vi "PowerSupplyModule.vi"(8 "error in (no error)":errorcluster, 9 "Shutdown Event":refnum<user-event>, 10 "Config":T1, 11 "ModuleID":string) -> (0 "error out":errorcluster)   [LabVIEW 2020, in "PowerSupply.lvlib"]
uses:
  PowerSupply.lvlib
  <vilib>/Utility/Data Type/Type Definitions/Data Type.ctl
  <vilib>/Utility/Data Type/NI_Data Type.lvlib
  eac3c09b-8ce1-4b18-8db3-0e6b686db002.vi
  <vilib>/Tag Engine/Types/SetRequest Cluster.ctl
  <vilib>/Tag Engine/Tag Engine Core.lvlib
  5bc3bb94-1071-4bc4-bea8-59b69d9a0ea3.vi
  2c36721a-ae4d-497d-865d-af4d970190ac.vi
  e0a74cc3-df72-4da2-81c8-b90a0d719853.vi
  32760def-be6c-40d5-9cdc-91618a22e337.vi
  fa7b8413-0d77-4427-8bf4-75f68590801f.vi
  674e74a0-18a0-4cb1-b513-5d1b134eea45.vi
  <vilib>/Tag Engine/Tag/Tag.lvclass
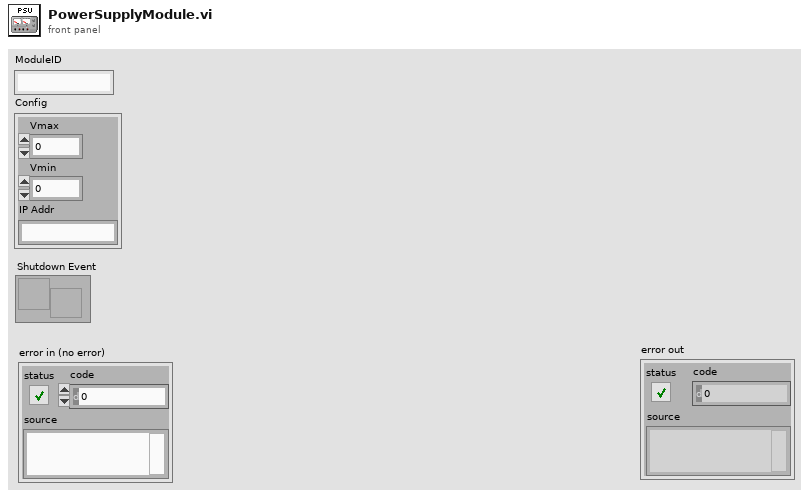
[diagram p1: front panel]
types:
  T1 = cluster{"Vmax":dbl, "Vmin":dbl, "IP Addr":string}
  T2 = cluster{"Config":cluster{"Vmax":dbl, "Vmin":dbl, "IP Addr":string}, "Tag Refs":cluster{"VOLT_SV":refnum<data-value>, "VOLT_PV":refnum<data-value>, "CURR_PV":refnum<data-value>, "OUTPUT_EN":refnum<data-value>}}
  T3 = cluster{"VOLT_SV":refnum<user-event>, "OUTPUT_EN":refnum<user-event>}
  T4 = cluster{"VOLT_SV":refnum<data-value>, "VOLT_PV":refnum<data-value>, "CURR_PV":refnum<data-value>, "OUTPUT_EN":refnum<data-value>}
  T5 = cluster{"Req Value":variant, "Callback":refnum<notifier>}
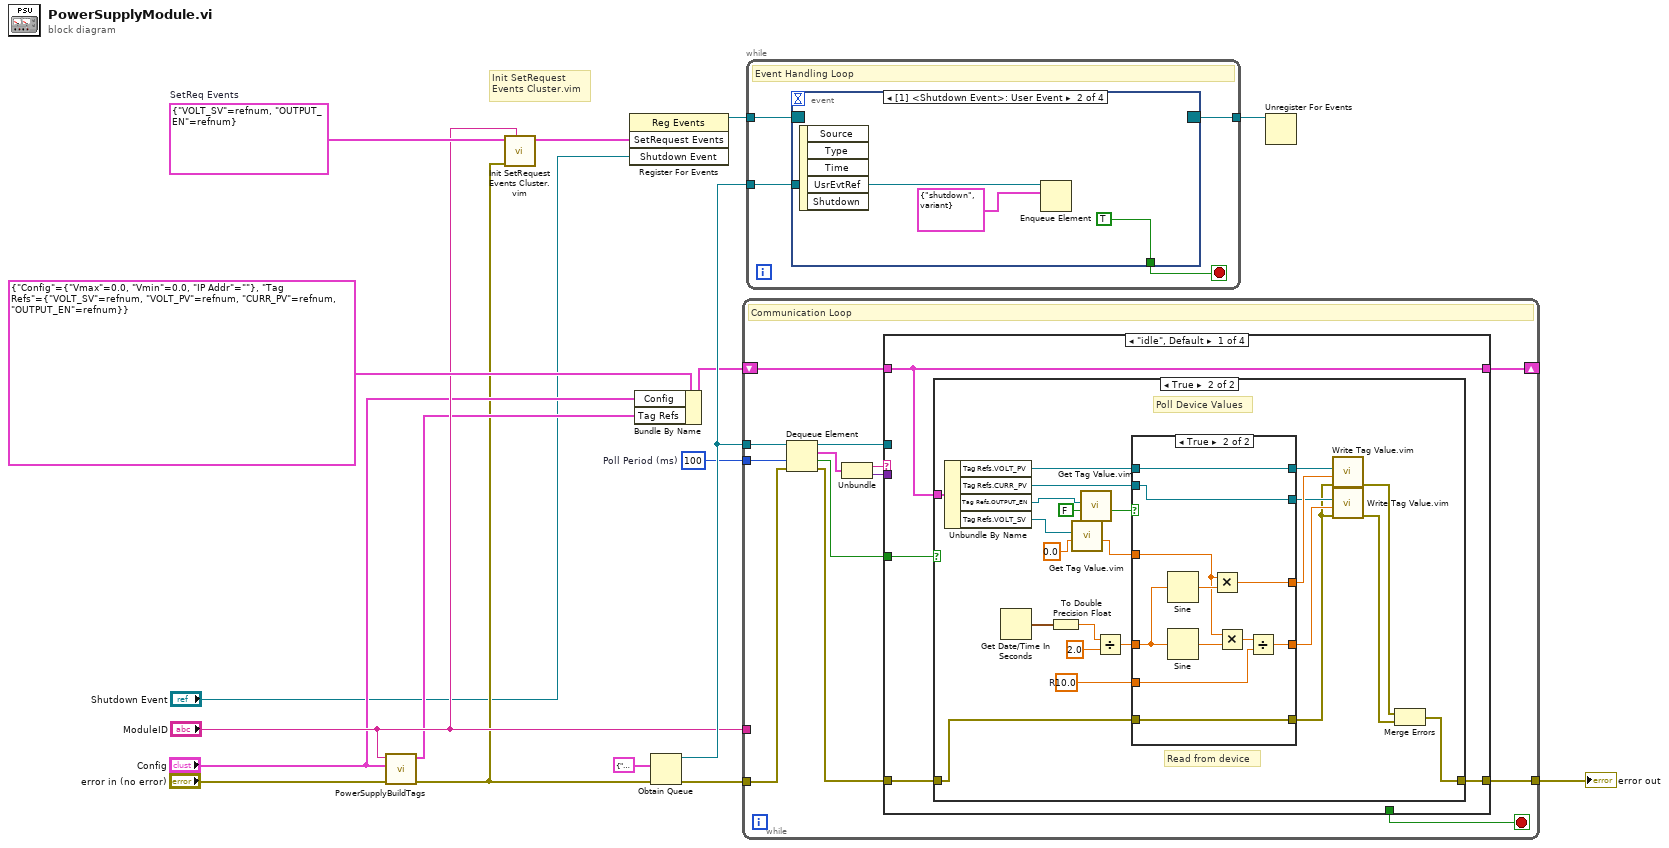
[diagram p0: block diagram]
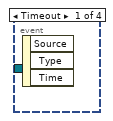
[diagram p2: hidden frame]
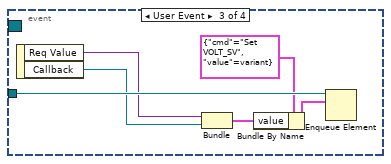
[diagram p3: hidden frame]
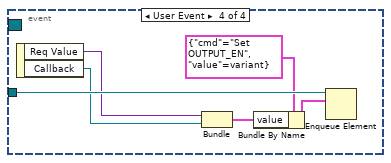
[diagram p4: hidden frame]
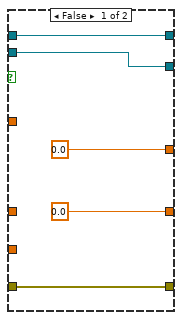
[diagram p6: hidden frame]
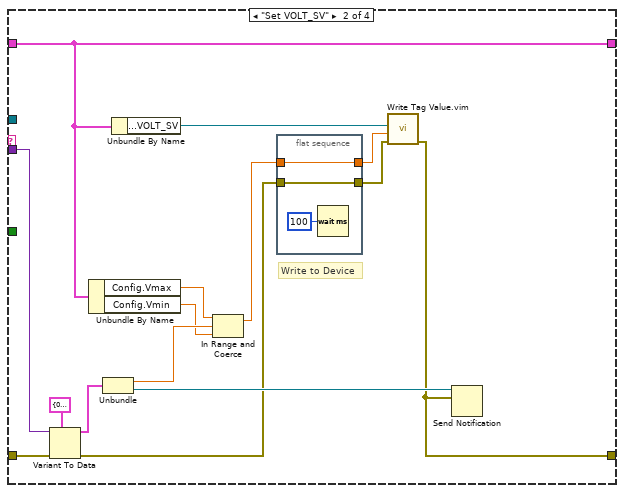
[diagram p7: hidden frame]
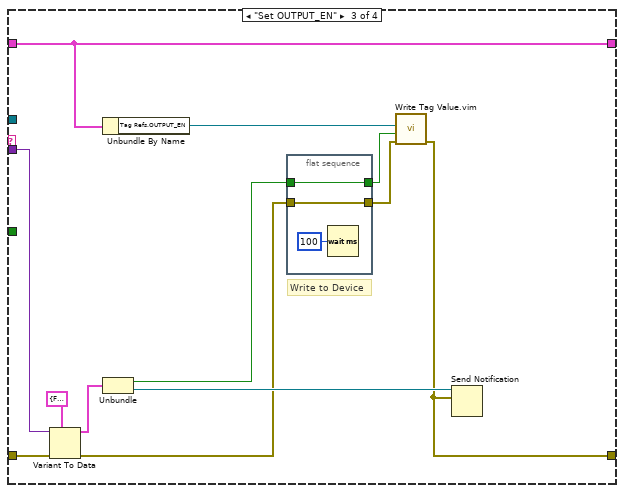
[diagram p8: hidden frame]
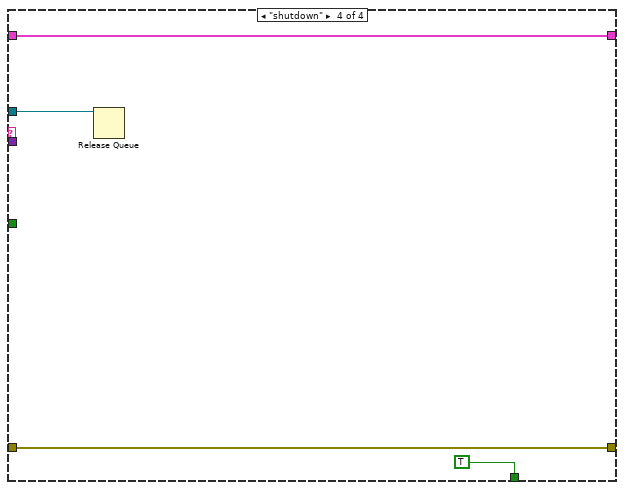
[diagram p9: hidden frame]
diagram:
  w2 = 100  # Poll Period (ms)
  w15 = T3 {"VOLT_SV"=refnum, "OUTPUT_EN"=refnum}  # SetReq Events
  # "Init SetRequest\nEvents Cluster.vim"
  n1 = call "PowerSupplyBuildTags.vi"("error in (no error)"="error in (no error)", "Config"="Config", "ModuleID"="ModuleID") -> ("error out"=w5:errorcluster, "Tag Refs"=w6:T4)  [unwired: 7 in]
  n2 = call "Init SetRequest Events Cluster.vim"("Namespace"="ModuleID", "error in (no error)"=w5, "SetRequest Events in"=w15) -> ("SetRequest Events"=w14:T3)  [unwired: 7 in, 1 out]
  n3 = register-events(w14, "Shutdown Event") -> (reference out=w16:refnum<event-registration>)  [unwired: 2 in, 1 out]
  n4 = Bundle By Name(cluster=T2 {"Config"={"Vmax"=0.0, "Vmin"=0.0, "IP Addr"=""}, "Tag Refs"={"VOLT_SV"=refnum, "VOLT_PV"=refnum, "CURR_PV"=refnum, "OUTPUT_EN"=refnum}}, "Config"="Config", "Tag Refs"=w6) -> (w3:T2)
  n5 = Obtain Queue(element data type=cluster{"cmd":string, "value":variant} {"cmd"="", "value"=variant}, error in (no error)=w5) -> (queue out=w12:refnum<queue>, error out=w4:errorcluster)  [unwired: 3 in, 1 out]
  n6 = while {
    tunnel: "ModuleID" -> [_]
    tunnel: w4 -> [w30]
    shift-right: [w22] -> _
    shift-left: w3 -> [w29]
    tunnel: w12 -> [w26]
    tunnel: [w20] -> w11
    tunnel: w2 -> [w18]
    stop <- w21 stop-if-true
    # "Communication Loop"
    n7 = Dequeue Element(queue=w26, timeout in ms (-1)=w18, error in (no error)=w30) -> (queue out=w27:refnum<queue>, element=w25:cluster{"cmd":string, "value":variant}, timed out?=w19:bool, error out=w28:errorcluster)
    n8 = Unbundle(w25) -> ("cmd"=w24:string, "value"=w23:variant)
    n9 = case shown="\"idle\", Default" w24 {
      tunnel: w29 -> [w34 w82 w100 w111]
      tunnel: w28 -> [w32 w89 w104 w108]
      tunnel: w27 -> [_ _ _ w109]
      tunnel: w23 -> [_ w88 w103 _]
      tunnel: [w34 w82 w100 w111] -> w22
      tunnel: [_ _ _ TRUE] -> w21
      tunnel: [w31 w79 w97 w108] -> w20
      tunnel: w19 -> [w33 _ _ _]
      frame "idle", Default {
        n10 = case shown="True" w33 {
          tunnel: w34 -> [_ w58]
          tunnel: w32 -> [w35 w46]
          tunnel: [w35 w42] -> w31
          frame False {
          }
          frame True {
            w51 = 10.0  # R
            # "Read from device"
            # "Poll Device Values"
            n11 = Unbundle By Name(w58) -> ("Tag Refs.VOLT_PV"=w57:refnum<data-value>, "Tag Refs.CURR_PV"=w56:refnum<data-value>, "Tag Refs.OUTPUT_EN"=w37:refnum<data-value>, "Tag Refs.VOLT_SV"=w36:refnum<data-value>)
            n12 = Get Date/Time In Seconds() -> (seconds since 1Jan1904=w55:timestamp)
            n13 = To Double Precision Float(number=w55) -> (double precision float=w53:dbl)
            n14 = call "Get Tag Value.vim"("Default (Void)"=0.0 ("Value(s)"), "Tag Name(s)/Ref(s)"=w36) -> ("Value(s)"=w38:dbl)  [unwired: 6 in, 3 out]
            n15 = call "Get Tag Value.vim"("Default (Void)"=FALSE, "Tag Name(s)/Ref(s)"=w37) -> ("Value(s)"=w40:bool)  [unwired: 6 in, 3 out]
            n16 = Divide(x=w53, y=2.0) -> (x/y=w52:dbl)
            n17 = case shown="True" w40 {
              tunnel: w57 -> [w61 w68]
              tunnel: w56 -> [w60 w67]
              tunnel: w38 -> [_ w73]
              tunnel: w52 -> [_ w65]
              tunnel: w51 -> [_ w71]
              tunnel: [0.0 w70] -> w49
              tunnel: [0.0 w69] -> w47
              tunnel: [w61 w68] -> w50
              tunnel: [w60 w67] -> w48
              tunnel: w46 -> [w59 w66]
              tunnel: [w59 w66] -> w45
              frame False {
              }
              frame True {
                n18 = Sine(x=w65) -> (sin(x)=w74:dbl)
                n19 = Sine(x=w65) -> (sin(x)=w64:dbl)
                n20 = Multiply(x=w73, y=w74) -> (x*y=w70:dbl)
                n21 = Multiply(x=w73, y=w64) -> (x*y=w72:dbl)
                n22 = Divide(x=w72, y=w71) -> (x/y=w69:dbl)
              }
            }
            n23 = call "Write Tag Value.vim"("error in (no error)"=w45, "Value"=w49, "Tag Name(s)/Ref(s)"=w50) -> ("error out"=w44:errorcluster)  [unwired: 7 in, 1 out]
            n24 = call "Write Tag Value.vim"("error in (no error)"=w45, "Value"=w47, "Tag Name(s)/Ref(s)"=w48) -> ("error out"=w43:errorcluster)  [unwired: 7 in, 1 out]
            n25 = Merge Errors(w44, w43) -> (w42:errorcluster)
          }
        }
      }
      frame "Set VOLT_SV" {
        # "Write to Device"
        n26 = Variant To Data(error in=w89, type=cluster{dbl, "Callback":refnum<notifier>} {0.0, "Callback"=refnum}, Variant=w88) -> (data=w86:cluster{dbl, "Callback":refnum<notifier>}, error out=w77:errorcluster)
        n27 = Unbundle By Name(w82) -> ("Config.Vmax"=w84:dbl, "Config.Vmin"=w83:dbl)
        n28 = Unbundle(w86) -> (w85:dbl, "Callback"=w80:refnum<notifier>)
        n29 = Unbundle By Name(w82) -> ("Tag Refs.VOLT_SV"=w81:refnum<data-value>)
        n30 = In Range and Coerce(upper limit=w84, x=w85, lower limit=w83) -> (coerced(x)=w76:dbl)  [unwired: 1 out]
        n31 = flat-sequence {
          tunnel: [w92] -> w78
          tunnel: w77 -> [w92]
          tunnel: w76 -> [w91]
          tunnel: [w91] -> w75
          frame #0 {
            n32 = Wait (ms)(milliseconds to wait=u32 100) -> ()  [unwired: 1 out]
          }
        }
        n33 = call "Write Tag Value.vim"("error in (no error)"=w78, "Value"=w75, "Tag Name(s)/Ref(s)"=w81) -> ("error out"=w79:errorcluster)  [unwired: 7 in, 1 out]
        n34 = Send Notification(notification=w79, notifier=w80) -> ()  [unwired: 1 in, 2 out]
      }
      frame "Set OUTPUT_EN" {
        # "Write to Device"
        n35 = Variant To Data(error in=w104, type=cluster{bool, "Callback":refnum<notifier>} {FALSE, "Callback"=refnum}, Variant=w103) -> (data=w101:cluster{bool, "Callback":refnum<notifier>}, error out=w96:errorcluster)
        n36 = Unbundle By Name(w100) -> ("Tag Refs.OUTPUT_EN"=w99:refnum<data-value>)
        n37 = Unbundle(w101) -> (w95:bool, "Callback"=w98:refnum<notifier>)
        n38 = flat-sequence {
          tunnel: [w107] -> w93
          tunnel: w96 -> [w107]
          tunnel: w95 -> [w106]
          tunnel: [w106] -> w94
          frame #0 {
            n39 = Wait (ms)(milliseconds to wait=u32 100) -> ()  [unwired: 1 out]
          }
        }
        n40 = call "Write Tag Value.vim"("error in (no error)"=w93, "Value"=w94, "Tag Name(s)/Ref(s)"=w99) -> ("error out"=w97:errorcluster)  [unwired: 7 in, 1 out]
        n41 = Send Notification(notification=w97, notifier=w98) -> ()  [unwired: 1 in, 2 out]
      }
      frame "shutdown" {
        n42 = Release Queue(queue=w109) -> ()  [unwired: 2 in, 3 out]
      }
    }
  }
  "error out" <- w11
  n43 = while {
    tunnel: [w115] -> w17
    tunnel: w16 -> [w114]
    tunnel: w12 -> [w112]
    stop <- w113 stop-if-true
    # "Event Handling Loop"
    n44 = event shown="[1] <Shutdown Event>: User Event" {
      selector: w114 -> [_ _ _ _]
      dyn-events: [_ _ _ _] -> w115
      timeout: _ -> [_ _ _ _]
      tunnel: [_ TRUE _ _] -> w113
      tunnel: w112 -> [_ w117 w124 w130]
      event Timeout {
        n45 = event-data() -> ()  [unwired: 1 in, 3 out]
      }
      event User Event {
        n46 = event-data() -> ()  [unwired: 1 in, 5 out]
        n47 = Enqueue Element(queue=w117, element=cluster{"cmd":string, "value":variant} {"cmd"="shutdown", "value"=variant}) -> ()  [unwired: 2 in, 3 out]
      }
      event User Event {
        n48 = event-data() -> ("Req Value"=w121:variant, "Callback"=w120:refnum<notifier>)  [unwired: 1 in]
        n49 = Bundle("Req Value"=w121, "Callback"=w120) -> (w119:T5)  [unwired: 1 in]
        n50 = Bundle By Name(cluster=cluster{"cmd":string, "value":variant} {"cmd"="Set VOLT_SV", "value"=variant} ("element"), "value"=w119) -> (w122:cluster{"cmd":string, "value":variant})
        n51 = Enqueue Element(queue=w124, element=w122) -> ()  [unwired: 2 in, 3 out]
      }
      event User Event {
        n52 = event-data() -> ("Req Value"=w127:variant, "Callback"=w126:refnum<notifier>)  [unwired: 1 in]
        n53 = Bundle("Req Value"=w127, "Callback"=w126) -> (w125:T5)  [unwired: 1 in]
        n54 = Bundle By Name(cluster=cluster{"cmd":string, "value":variant} {"cmd"="Set OUTPUT_EN", "value"=variant} ("element"), "value"=w125) -> (w128:cluster{"cmd":string, "value":variant})
        n55 = Enqueue Element(queue=w130, element=w128) -> ()  [unwired: 2 in, 3 out]
      }
    }
  }
  n56 = Unregister For Events(event registration refnum=w17) -> ()  [unwired: 1 in, 1 out]
